vi "Read Refs.vi"(11 "Project Stuff in":refnum<class "Project Stuff.lvclass">) -> (2 "Refs":T1)   [LabVIEW 2025, in "_Shared.lvlib" / "Project Stuff.lvclass"]
uses:
  Project Stuff.lvclass
  Project Stuff.lvclass/Project Stuff.ctl
  VI.ctl
  Library.ctl
  Descendents.ctl
  Refs.ctl
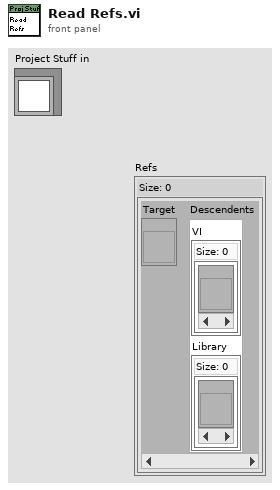
[diagram p1: front panel]
types:
  T1 = typedef "_Shared.lvlib/Project Stuff.lvclass/Refs.ctl" = map{refnum<vi>, T2}
  T2 = typedef "_Shared.lvlib/Project Stuff.lvclass/Descendents.ctl" = cluster{"VI":T3, "Library":T4}
  T3 = typedef "_Shared.lvlib/Project Stuff.lvclass/VI.ctl" = set{refnum<vi>}
  T4 = typedef "_Shared.lvlib/Project Stuff.lvclass/Library.ctl" = set{refnum<vi>}
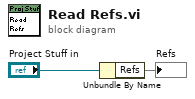
[diagram p0: block diagram]
diagram:
  n1 = Unbundle By Name("Project Stuff in") -> ("Refs"=→"Refs":T1)
